vi "Puckbot Main.vi"() -> ()   [LabVIEW 2019]
uses:
  SubVIs/Voter Info.ctl
  Vote Handler/Vote Result.ctl
  Vote Handler/Vote Status Update.ctl
  SubVIs/References.ctl
  <vilib>/MediaMongrels Ltd/Message Queue Helper/ctl_QMH_Message_Typedef.ctl
  SubVIs/Move Type.ctl
  Vote Handler/VoteMessage.ctl
  LINX-PCA9865 PWM/LINX-PCA9865 PWM.lvclass
  LINX-PCA9865 PWM/LINX-PCA9865 PWM.lvclass/LINX-PCA9865 PWM.ctl
  LINX-PCA9865 PWM/Write LINX Resource.vi
  LINX-PCA9865 PWM/Write I2C Slave Address (0x40).vi
  LINX-PCA9865 PWM/Write LINX I2C Channel.vi
  LINX-PCA9865 PWM/Read LINX Resource.vi
  <vilib>/MakerHub/LINX/Public/Utilities/Open Local.vi
  <vilib>/MediaMongrels Ltd/WebSockets/Sockets/VISA TCP Listener/VISA TCP Listener.lvclass
  <vilib>/MediaMongrels Ltd/WebSockets/WebSockets/WebSocket Server/WebSocket Server.lvclass
  <vilib>/MediaMongrels Ltd/Message Queue Helper/MessageQueueHelper.lvlib
  <vilib>/MakerHub/LINX/LMH-LINX.lvlib
panel:
  out "Frequency (Hz)":dbl
  out "Error":errorcluster
  in  "stop":bool
  out "Drives Enabled?":bool
  out "Status":T1
  out "Time Remaining":dbl format="%<%H:%M:%S%2u>t"
  out "Vote Count":T2[](array[typedef])
  out "Voters":cluster{"VoterID":i32, "VoterInfo":T3}[](array[cluster])
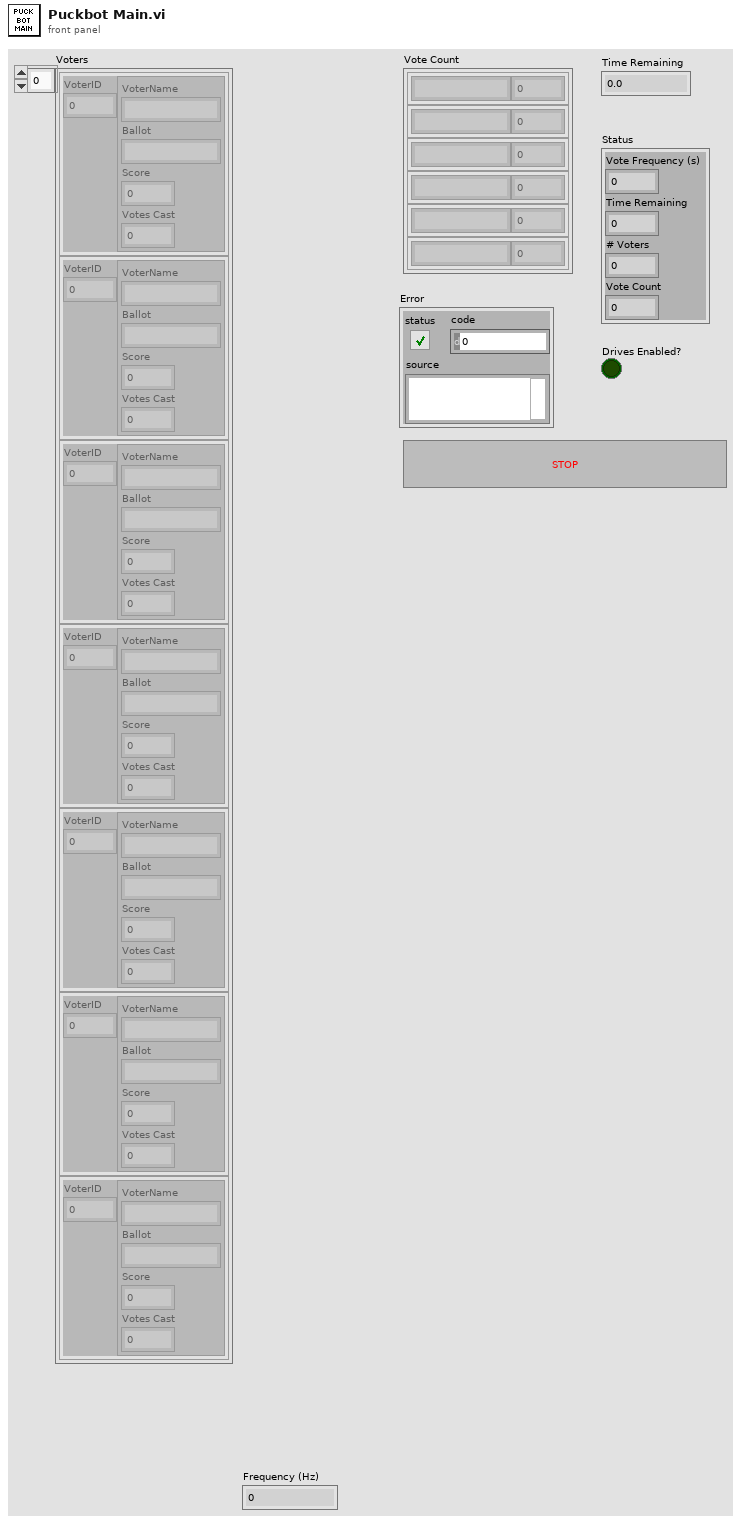
[diagram p1: front panel]
types:
  T1 = typedef "Vote Status Update.ctl" = cluster{"Vote Frequency (s)":dbl, "Time Remaining":dbl, "# Voters":i32, "Vote Count":i32}
  T2 = typedef "Vote Result.ctl" = cluster{"Vote":string, "Count":i32}
  T3 = typedef "Voter Info.ctl" = cluster{"VoterName":string, "Ballot":string, "Score":i32, "Votes Cast":i32}
  T4 = typedef "Move Type.ctl" = cluster{"Option":string, "Left":dbl, "Right":dbl, "Duration":dbl}
  T5 = typedef "References.ctl" = cluster{"Vote Queue":refnum<queue>, "Message Event":refnum<user-event>}
  T6 = typedef "LMH-LINX.lvlib/LINX Ref.ctl" = cluster{"IO":T7, "Interface":T8, "LINX Device Config":T9}
  T7 = typedef "LMH-LINX.lvlib/Platform.ctl" = enum16{"Remote", "Local"}
  T8 = typedef "LMH-LINX.lvlib/Interface.ctl" = enum16{"Serial", "TCP"}
  T9 = typedef "LMH-LINX.lvlib/Device.lvlib/LINX Device Config.ctl" = cluster{"Interface":T8, "COM Port":refnum<visa-resource-name>, "TCP Configuration":T10, "Device Family":u8, "Device ID":u8, "Device Name":string, "TCP Ref":refnum<k5>, "Channels":T11}
  T10 = typedef "LMH-LINX.lvlib/Device.lvlib/TCP Config.ctl" = cluster{"IP Address":string, "Port":u16}
  T11 = typedef "LMH-LINX.lvlib/Channels.ctl" = cluster{"DI":u8[], "DO":u8[], "AI":u8[], "AO":u8[], "PWM":u8[], "QE":u8[], "UART":u8[], "I2C 2":u8[], "SPI":u8[], "CAN":u8[], "Servo":u8[], "AI Ref (V)":dbl, "AI Resolution (Bits)":u8, "AO Ref (V)":dbl, "AO Resolution (Bits)":u8}
  T12 = enum16{"LED/PWM00", "LED/PWM01", "LED/PWM02", "LED/PWM03", "LED/PWM04", "LED/PWM05", "LED/PWM06", "LED/PWM07", "LED/PWM08", "LED/PWM09", "LED/PWM10", "LED/PWM11", "LED/PWM12", "LED/PWM13", "LED/PWM14", "LED/PWM15"}[]
  T13 = typedef "VoteMessage.ctl" = cluster{"VoterID":i32, "VoterInfo":T3}
  T14 = typedef "Scoreboard Entry.ctl" = cluster{"VoterName":string, "Score":i32}
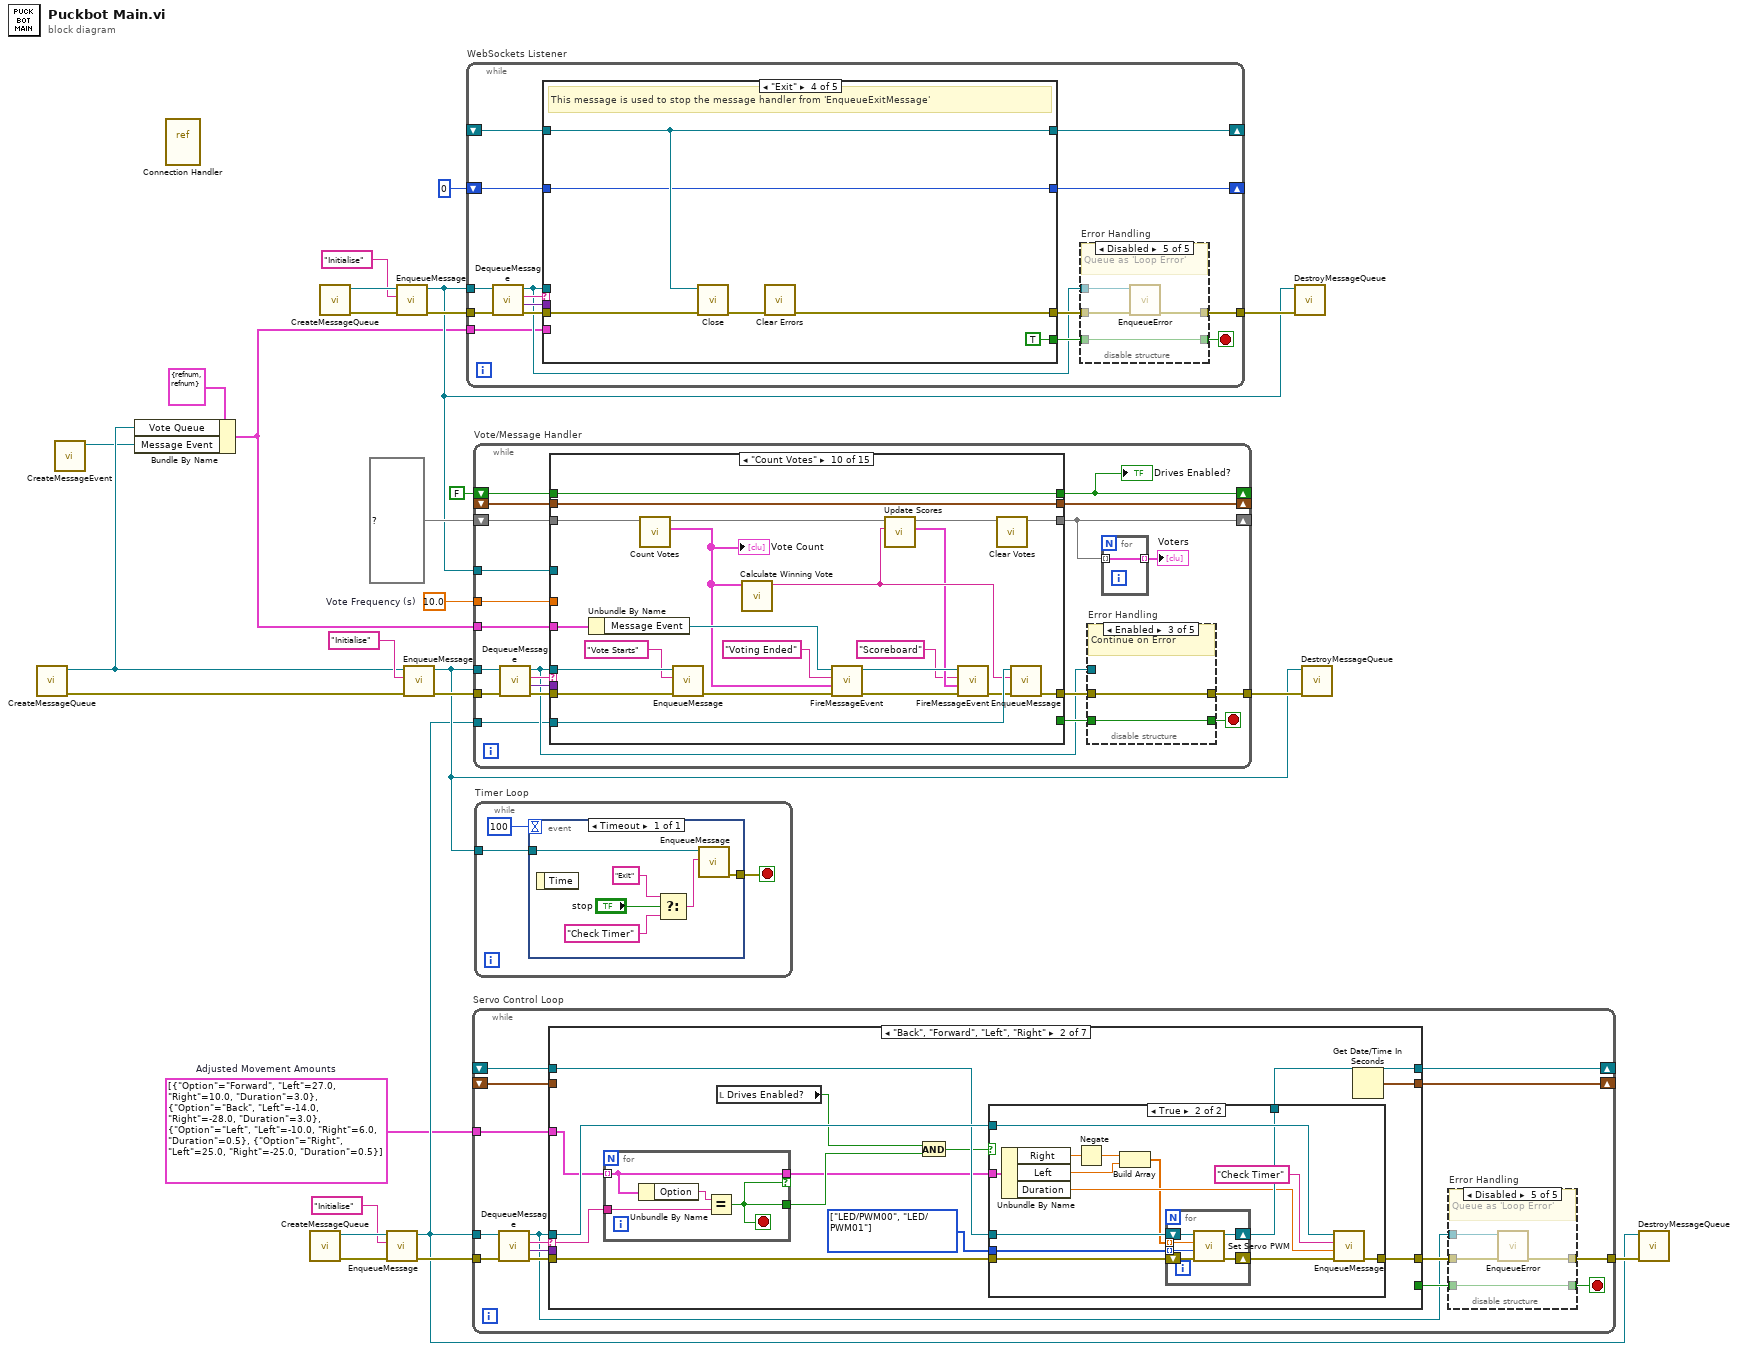
[diagram p0: block diagram]
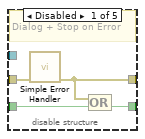
[diagram p2: hidden frame]
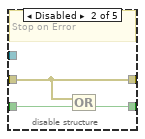
[diagram p3: hidden frame]
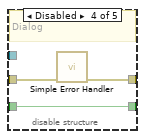
[diagram p5: hidden frame]
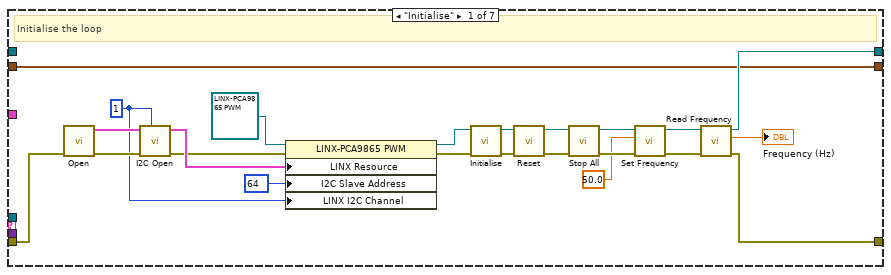
[diagram p6: hidden frame]
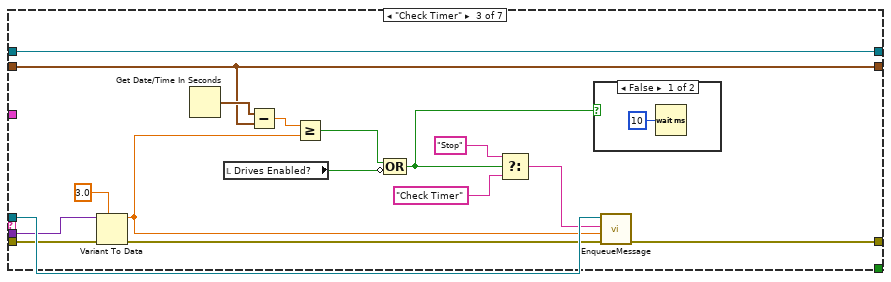
[diagram p8: hidden frame]
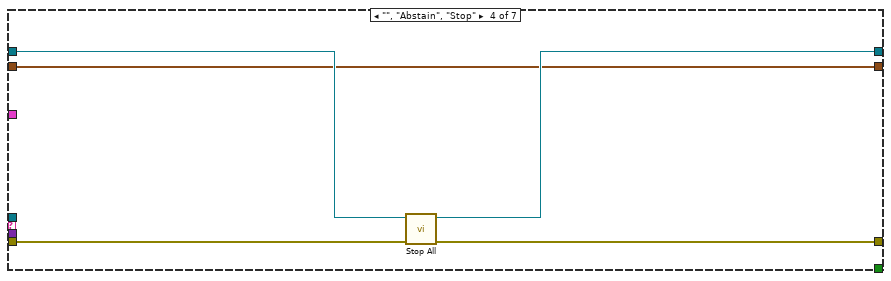
[diagram p10: hidden frame]
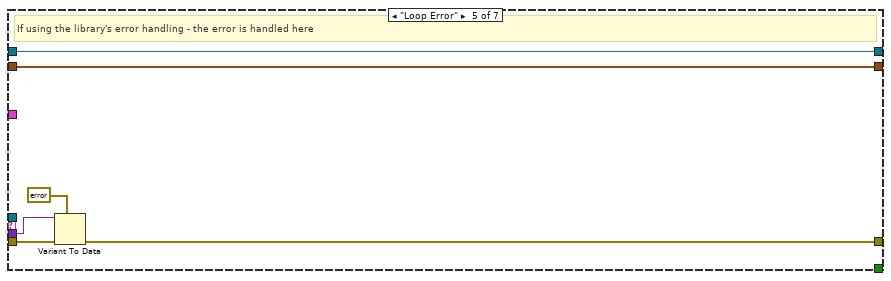
[diagram p11: hidden frame]
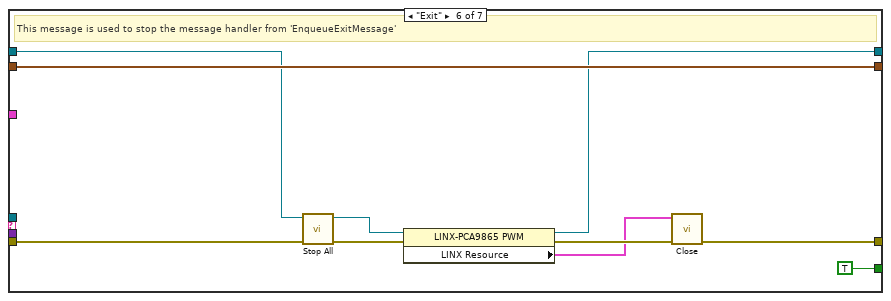
[diagram p12: hidden frame]
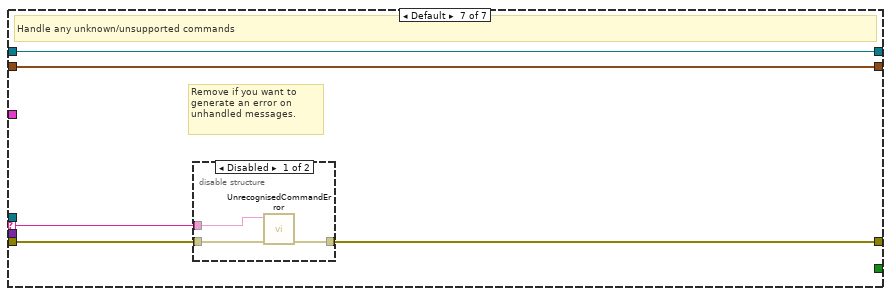
[diagram p13: hidden frame]
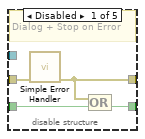
[diagram p15: hidden frame]
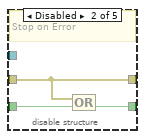
[diagram p16: hidden frame]
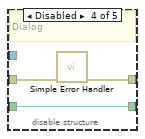
[diagram p17: hidden frame]
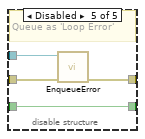
[diagram p18: hidden frame]
diagram:
  w1 = T4[] [{"Option"="Forward", "Left"=27.0, "Right"=10.0, "Duration"=3.0}, {"Option"="Back", "Left"=-14.0, "Right"=-28.0, "Duration"=3.0}, {"Option"="Left", "Left"=-10.0, "Right"=6.0, "Duration"=0.5}, {"Option"="Right", "Left"=25.0, "Right"=-25.0, "Duration"=0.5}]  # Adjusted Movement Amounts
  w14 = 10.0  # Vote Frequency (s)
  n1 = call <vilib>:"CreateMessageQueue.vi"() -> ("error out"=w17:errorcluster, "queue out"=w12:refnum<queue>)  [unwired: 9 in, 1 out]
  n2 = call <vilib>:"CreateMessageEvent.vi"() -> ("Message Event"=w11:refnum<user-event>)  [unwired: 10 in, 1 out]
  n3 = Bundle By Name(cluster=T5 {"Vote Queue"=refnum, "Message Event"=refnum} ("output cluster"), "Vote Queue"=w12, "Message Event"=w11) -> (w9:T5)
  n4 = vi-ref "Connection Handler.vi"() -> ()  [unwired: 1 out]
  n5 = call <vilib>:"CreateMessageQueue.vi"() -> ("error out"=w3:errorcluster, "queue out"=w5:refnum<queue>)  [unwired: 9 in, 1 out]
  n6 = call <vilib>:"CreateMessageQueue.vi"() -> ("error out"=w22:errorcluster, "queue out"=w24:refnum<queue>)  [unwired: 9 in, 1 out]
  n7 = call <vilib>:"EnqueueMessage.vi"("error in (no error)"=w3, "Command"="Initialise", "Message Queue in"=w5) -> ("error out"=w6:errorcluster, "Message Queue out"=w2:refnum<queue>)  [unwired: 6 in, 1 out]
  n8 = call <vilib>:"EnqueueMessage.vi"("error in (no error)"=w22, "Command"="Initialise", "Message Queue in"=w24) -> ("error out"=w25:errorcluster, "Message Queue out"=w10:refnum<queue>)  [unwired: 6 in, 1 out]
  n9 = call <vilib>:"EnqueueMessage.vi"("error in (no error)"=w17, "Command"="Initialise", "Message Queue in"=w12) -> ("error out"=w19:errorcluster, "Message Queue out"=w15:refnum<queue>)  [unwired: 6 in, 1 out]
  n10 = while "WebSockets Listener" {
    tunnel: w25 -> [w41]
    tunnel: w10 -> [w40]
    tunnel: [w33] -> w26
    shift-right: [w31] -> _
    shift-left: _ -> [w30]
    tunnel: w9 -> [w29]
    shift-right: [w27] -> _
    shift-left: 0 -> [w28]
    stop <- w35 stop-if-true
    n11 = call <vilib>:"DequeueMessage.vi"("error in (no error)"=w41, "Message Queue in"=w40) -> ("error out"=w37:errorcluster, "Data"=w38:variant, "Command"=w39:string, "Message Queue out"=w32:refnum<queue>)  [unwired: 5 in, 1 out]
    n12 = case shown="\"Exit\"" w39 {
      selector: w39 -> [_ _ _ _ w130]
      tunnel: w38 -> [_ _ w120 _ _]
      tunnel: w37 -> [w65 w84 w121 w126 w132]
      tunnel: w32 -> [w60 w78 _ _ _]
      tunnel: [w61 w79 w112 w125 w131] -> w36
      tunnel: [_ _ _ TRUE _] -> w34
      tunnel: [w66 w82 w118 w124 w129] -> w31
      tunnel: w30 -> [w64 w83 w118 w124 w129]
      tunnel: w29 -> [_ w77 w111 _ _]
      tunnel: w28 -> [w58 w76 w117 w123 w128]
      tunnel: [w58 w75 w117 w123 w128] -> w27
      frame "Initialise" {
        # "Initialise the loop"
        n13 = call-dynamic <vilib>:"Close.vi"("error in (no error)"=w65, "VISA TCP Listener in"=w64) -> ("error out"=w59:errorcluster)  [unwired: 9 in]
        n14 = call <vilib>:"Clear Errors.vi"("error in (no error)"=w59) -> ("error out"=w63:errorcluster)  [unwired: 5 in, 1 out]
        n15 = call <vilib>:"New VISA TCP Listener.vi"("error in (no error)"=w63) -> ("error out"=w68:errorcluster, "VISA TCP Listener out"=w67:refnum<class "VISA TCP Listener.lvclass">)  [unwired: 9 in]
        n16 = call-dynamic "Create Listener.vi"("error in (no error)"=w68, "Port"=u16 6123, "VISA TCP Listener in"=w67) -> ("error out"=w62:errorcluster, "VISA TCP Listener out"=w66:refnum<class "VISA TCP Listener.lvclass">)  [unwired: 7 in]
        n17 = case shown="No Error" w62 {
          selector: w62 -> [w73 w74]
          tunnel: [w72 w74] -> w61
          tunnel: w60 -> [w71 _]
          frame No Error {
            n18 = call <vilib>:"EnqueueMessage.vi"("error in (no error)"=w73, "Command"="Listen", "Message Queue in"=w71) -> ("error out"=w72:errorcluster)  [unwired: 6 in, 2 out]
          }
          frame Error {
          }
        }
      }
      frame "Listen" {
        n19 = call-dynamic "Wait on Listener.vi"("error in (no error)"=w84, "timeout ms (5000)"=200, "VISA TCP Listener in"=w83) -> ("error out"=w81:errorcluster, "Socket out"=w80:refnum<class "Socket.lvclass">, "VISA TCP Listener out"=w82:refnum<class "VISA TCP Listener.lvclass">)  [unwired: 6 in]
        n20 = case shown="No Error" w81 {
          selector: w81 -> [w96 w102 w108]
          tunnel: w80 -> [w97 _ _]
          tunnel: [w90 w102 w106] -> w79
          tunnel: w78 -> [w92 _ w105]
          tunnel: w77 -> [w88 _ _]
          tunnel: w76 -> [w87 w100 w103]
          tunnel: [w86 w100 w103] -> w75
          frame No Error {
            n21 = call <vilib>:"New Server from Socket.vi"("error in (no error)"=w96, "Socket"=w97) -> ("error out"=w98:errorcluster, "WebSocket Server out"=w99:refnum<class "WebSocket Server.lvclass">)  [unwired: 8 in]
            n22 = call-dynamic "Handshake.vi"("error in (no error)"=w98, "WebSocket Connection in"=w99) -> ("error out"=w95:errorcluster, "WebSocket Connection out"=w94:refnum<class "WebSocket Server.lvclass">)  [unwired: 8 in]
            n23 = call "Launch Connection Handler.vi"("error in (no error)"=w95, "ConnectionID"=w87, "References in"=w88, "WebSocket Connection in"=w94) -> ("error out"=w93:errorcluster)  [unwired: 7 in]
            n24 = call <vilib>:"EnqueueMessage.vi"("Command"="Listen", "Message Queue in"=w92) -> ("error out"=w89:errorcluster)  [unwired: 7 in, 2 out]
            n25 = Increment(x=w87) -> (x+1=w86:i32)
            n26 = Merge Errors(w93, w89) -> (w90:errorcluster)
          }
          frame Default {
            n27 = Wait (ms)(milliseconds to wait=u32 10) -> ()  [unwired: 1 out]
          }
          frame Error {
            n28 = call <vilib>:"Clear Errors.vi"("error in (no error)"=w108) -> ("error out"=w107:errorcluster)  [unwired: 5 in, 1 out]
            n29 = call <vilib>:"EnqueueMessage.vi"("error in (no error)"=w107, "Command"="Listen", "Message Queue in"=w105) -> ("error out"=w106:errorcluster)  [unwired: 6 in, 2 out]
          }
        }
      }
      frame "Loop Error" {
        # "If using the library's error handling - the error is handled here"
        n30 = Variant To Data(error in=w121, type=errorcluster {"status"=FALSE, "code"=0, "source"=""} ("error constant"), Variant=w120) -> (data=w114:errorcluster, error out=w116:errorcluster)
        n31 = Unbundle By Name(w111) -> ("Vote Queue"=w110:refnum<queue>)
        n32 = Merge Errors(w114, w116) -> (w115:errorcluster)
        n33 = call <vilib>:"EnqueueError.vi"("Source"="Listener", "error in (no error)"=w115, "Message Queue in"=w110) -> ("error out"=w113:errorcluster)  [unwired: 8 in]
        n34 = call <vilib>:"Clear Errors.vi"("error in (no error)"=w113) -> ("error out"=w112:errorcluster)  [unwired: 5 in, 1 out]
      }
      frame "Exit" {
        # "This message is used to stop the message handler from 'EnqueueExitMessage'"
        n35 = call-dynamic <vilib>:"Close.vi"("error in (no error)"=w126, "VISA TCP Listener in"=w124) -> ("error out"=w122:errorcluster)  [unwired: 9 in]
        n36 = call <vilib>:"Clear Errors.vi"("error in (no error)"=w122) -> ("error out"=w125:errorcluster)  [unwired: 5 in, 1 out]
      }
      frame Default {
        # "Remove if you want to generate an error on unhandled messages."
        # "Handle any unknown/unsupported commands"
        n37 = disable-structure shown="Disabled" {
          disable-tunnel: w132 -> [w134 w136]
          disable-tunnel: [w135 w136] -> w131
          disable-tunnel: w130 -> [w133 _]
          frame Disabled {
            n38 = call <vilib>:"UnrecognisedCommandError.vi"("error in (no error)"=w134, "Command"=w133) -> ("error out"=w135:errorcluster)  [unwired: 9 in]
          }
          frame Enabled {
          }
        }
      }
    }
    n39 = disable-structure "Error Handling" shown="Disabled" {
      disable-tunnel: w34 -> [w45 w48 w49 w52 w55]
      disable-tunnel: w36 -> [w44 w46 w50 w53 w57]
      disable-tunnel: [w43 w47 w49 w52 w55] -> w35
      disable-tunnel: [w42 w46 w50 w51 w56] -> w33
      disable-tunnel: w32 -> [_ _ _ _ w54]
      frame Disabled {
        # "Dialog + Stop on Error"
        n40 = call <vilib>:"Simple Error Handler.vi"("error in (no error)"=w44) -> ("error out"=w42:errorcluster)  [unwired: 4 in, 4 out]
        n41 = Compound Arithmetic op=OR(w42, w45) -> (w43:bool)
      }
      frame Disabled {
        # "Stop on Error"
        n42 = Compound Arithmetic op=OR(w46, w48) -> (w47:bool)
      }
      frame Enabled {
        # "Continue on Error"
      }
      frame Disabled {
        # "Dialog"
        n43 = call <vilib>:"Simple Error Handler.vi"("error in (no error)"=w53) -> ("error out"=w51:errorcluster)  [unwired: 4 in, 4 out]
      }
      frame Disabled {
        # "Queue as 'Loop Error'"
        n44 = call <vilib>:"EnqueueError.vi"("error in (no error)"=w57, "Message Queue in"=w54) -> ("error out"=w56:errorcluster)  [unwired: 9 in]
      }
    }
  }
  n45 = while "Servo Control Loop" {
    tunnel: w6 -> [w151]
    tunnel: w2 -> [w150]
    tunnel: [w143] -> w7
    shift-right: [w141] -> _
    shift-left: _ -> [w140]
    shift-right: [w139] -> _
    shift-left: _ -> [w138]
    tunnel: w1 -> [w137]
    stop <- w145 stop-if-true
    n46 = call <vilib>:"DequeueMessage.vi"("error in (no error)"=w151, "Message Queue in"=w150) -> ("error out"=w147:errorcluster, "Data"=w148:variant, "Command"=w149:string, "Message Queue out"=w142:refnum<queue>)  [unwired: 5 in, 1 out]
    n47 = case shown="\"Back\", \"Forward\", \"Left\", \"Right\"" w149 {
      selector: w149 -> [_ w193 _ _ _ _ w271]
      tunnel: w148 -> [_ _ w232 _ w256 _ _]
      tunnel: w147 -> [w170 w199 w239 w252 w258 w266 w273]
      tunnel: w142 -> [_ w201 w240 _ _ _ _]
      tunnel: [w169 w202 w238 w251 w257 w260 w272] -> w146
      tunnel: [_ _ _ _ _ TRUE _] -> w144
      tunnel: [w171 w197 w246 w249 w254 w263 w270] -> w141
      tunnel: w140 -> [_ w198 w246 w250 w254 w265 w270]
      tunnel: [w168 w203 w244 w248 w253 w267 w269] -> w139
      tunnel: w138 -> [w168 _ w244 w248 w253 w267 w269]
      tunnel: w137 -> [_ w192 _ _ _ _ _]
      frame "Initialise" {
        w174 = u8 1 ("I2C Channel")
        # "Initialise the loop"
        n48 = call-poly <vilib>:"Open.vi"("Error In"=w170) -> ("Error Out"=w177:errorcluster, "LINX Resource"=w176:T6)  [unwired: 8 in, 1 out]
        n49 = call <vilib>:"I2C Open.vi"("I2C Channel (0)"=w174, "Error In"=w177, "LINX Resource"=w176) -> ("Error Out"=w178:errorcluster, "LINX Resource"=w179:T6)  [unwired: 7 in]
        n50 = property class="LINX-PCA9865 PWM"(reference=refnum<class "LINX-PCA9865 PWM.lvclass"> refnum ("LINX-PCA9865 PWM.lvclass"), error in=w178, "LINX Resource"=w179, "I2C Slave Address"=u8 64 ("I2C Slave Address (0)"), "LINX I2C Channel"=w174) -> (reference out=w181:refnum<class "LINX-PCA9865 PWM.lvclass">, error out=w180:errorcluster)
        n51 = call-dynamic "Initialise.vi"("error in (no error)"=w180, "PWM in"=w181) -> ("error out"=w184:errorcluster, "PWM out"=w183:refnum<class "LINX-PCA9865 PWM.lvclass">)  [unwired: 8 in]
        n52 = call-dynamic "Reset.vi"("error in (no error)"=w184, "PWM in"=w183) -> ("error out"=w185:errorcluster, "PWM out"=w186:refnum<class "LINX-PCA9865 PWM.lvclass">)  [unwired: 8 in]
        n53 = call-dynamic "Stop All.vi"("error in (no error)"=w185, "LINX-PCA9865 PWM in"=w186) -> ("error out"=w189:errorcluster, "LINX-PCA9865 PWM out"=w190:refnum<class "LINX-PCA9865 PWM.lvclass">)  [unwired: 8 in]
        n54 = call-dynamic "Set Frequency.vi"("error in (no error)"=w189, "Frequency (1000Hz)"=50.0, "PWM in"=w190) -> ("error out"=w187:errorcluster, "PWM out"=w188:refnum<class "LINX-PCA9865 PWM.lvclass">)  [unwired: 7 in]
        n55 = call-dynamic "Read Frequency.vi"("error in (no error)"=w187, "PWM in"=w188) -> ("error out"=w169:errorcluster, "Frequency (Hz)"=→"Frequency (Hz)":dbl, "PWM out"=w171:refnum<class "LINX-PCA9865 PWM.lvclass">)  [unwired: 7 in]
      }
      frame "Back", "Forward", "Left", "Right" {
        w200 = T12 [enum."LED/PWM00", enum."LED/PWM01"] items=["LED/PWM00", "LED/PWM01", "LED/PWM02", "LED/PWM03", "LED/PWM04", "LED/PWM05", "LED/PWM06", "LED/PWM07", "LED/PWM08", "LED/PWM09", "LED/PWM10", "LED/PWM11", "LED/PWM12", "LED/PWM13", "LED/PWM14", "LED/PWM15"] ("LEDn (PWM channel)")
        n56 = for {
          tunnel: w192 -> [w206] mode=indexing
          tunnel: [w206] -> w191 if=w204
          tunnel: w193 -> [w205]
          tunnel: [w204] -> w195
          stop <- w204 stop-if-true
          n57 = Unbundle By Name(w206) -> ("Option"=w207:string)
          n58 = Equal?(x=w207, y=w205) -> (x = y?=w204:bool)
        }
        n59 = local read "Drives Enabled?"() -> (w196:bool)
        n60 = And(x=w196, y=w195) -> (x .and. y?=w194:bool)
        n61 = case shown="True" w194 {
          tunnel: [w208 w223] -> w202
          tunnel: w201 -> [_ w222]
          tunnel: w200 -> [_ w220]
          tunnel: w199 -> [w208 w219]
          tunnel: w198 -> [w209 w217]
          tunnel: [w209 w216] -> w197
          tunnel: w191 -> [_ w211]
          frame False {
          }
          frame True {
            n62 = Unbundle By Name(w211) -> ("Right"=w213:dbl, "Left"=w214:dbl, "Duration"=w212:dbl)
            n63 = Negate(x=w213) -> (-x=w215:dbl)
            n64 = Build Array(w215, w214) -> (w210:dbl[])
            n65 = for {
              tunnel: w210 -> [w226] mode=indexing
              tunnel: w220 -> [w225] mode=indexing
              shift-right: [w227] -> w216
              shift-left: w217 -> [w229]
              shift-right: [w228] -> w218
              shift-left: w219 -> [w224]
              n66 = call "Set Servo PWM.vi"("error in (no error)"=w224, "LEDn (PWM channel)"=w225, "Servo Speed (-100 to 100%)"=w226, "LINX-PCA9865 PWM in"=w229) -> ("error out"=w228:errorcluster, "LINX-PCA9865 PWM out"=w227:refnum<class "LINX-PCA9865 PWM.lvclass">)  [unwired: 6 in]
            }
            n67 = call <vilib>:"EnqueueMessage.vi"("error in (no error)"=w218, "Data"=w212, "Command"="Check Timer", "Message Queue in"=w222) -> ("error out"=w223:errorcluster)  [unwired: 5 in, 2 out]
          }
        }
        n68 = Get Date/Time In Seconds() -> (seconds since 1Jan1904=w203:timestamp)
      }
      frame "Check Timer" {
        n69 = Variant To Data(error in=w239, type=3.0 ("y"), Variant=w232) -> (data=w230:dbl, error out=w233:errorcluster)
        n70 = Get Date/Time In Seconds() -> (seconds since 1Jan1904=w245:timestamp)
        n71 = local read "Drives Enabled?"() -> (w241:bool)
        n72 = Subtract(x=w245, y=w244) -> (x-y=w243:dbl)
        n73 = Greater Or Equal?(x=w243, y=w230) -> (x >= y?=w242:bool)
        n74 = Compound Arithmetic op=OR(w242, invert w241) -> (w234:bool)
        n75 = Select(t="Stop", s=w234, f="Check Timer") -> (s? t:f=w235:string)
        n76 = case shown="False" w234 {
          frame False {
            n77 = Wait (ms)(milliseconds to wait=u32 10) -> ()  [unwired: 1 out]
          }
          frame True {
          }
        }
        n78 = call <vilib>:"EnqueueMessage.vi"("error in (no error)"=w233, "Data"=w230, "Command"=w235, "Message Queue in"=w240) -> ("error out"=w238:errorcluster)  [unwired: 5 in, 2 out]
      }
      frame "", "Abstain", "Stop" {
        n79 = call-dynamic "Stop All.vi"("error in (no error)"=w252, "LINX-PCA9865 PWM in"=w250) -> ("error out"=w251:errorcluster, "LINX-PCA9865 PWM out"=w249:refnum<class "LINX-PCA9865 PWM.lvclass">)  [unwired: 8 in]
      }
      frame "Loop Error" {
        # "If using the library's error handling - the error is handled here"
        n80 = Variant To Data(error in=w258, type=errorcluster {"status"=FALSE, "code"=0, "source"=""} ("error constant"), Variant=w256) -> (error out=w257:errorcluster)  [unwired: 1 out]
      }
      frame "Exit" {
        # "This message is used to stop the message handler from 'EnqueueExitMessage'"
        n81 = call-dynamic "Stop All.vi"("error in (no error)"=w266, "LINX-PCA9865 PWM in"=w265) -> ("error out"=w262:errorcluster, "LINX-PCA9865 PWM out"=w264:refnum<class "LINX-PCA9865 PWM.lvclass">)  [unwired: 8 in]
        n82 = property class="LINX-PCA9865 PWM"(reference=w264, error in=w262) -> (reference out=w263:refnum<class "LINX-PCA9865 PWM.lvclass">, error out=w261:errorcluster, "LINX Resource"=w259:T6)
        n83 = call <vilib>:"Close.vi"("Error In"=w261, "LINX Resource"=w259) -> ("Error Out"=w260:errorcluster)  [unwired: 9 in]
      }
      frame Default {
        # "Remove if you want to generate an error on unhandled messages."
        # "Handle any unknown/unsupported commands"
        n84 = disable-structure shown="Disabled" {
          disable-tunnel: w273 -> [w275 w277]
          disable-tunnel: [w276 w277] -> w272
          disable-tunnel: w271 -> [w274 _]
          frame Disabled {
            n85 = call <vilib>:"UnrecognisedCommandError.vi"("error in (no error)"=w275, "Command"=w274) -> ("error out"=w276:errorcluster)  [unwired: 9 in]
          }
          frame Enabled {
          }
        }
      }
    }
    n86 = disable-structure "Error Handling" shown="Disabled" {
      disable-tunnel: w144 -> [w155 w158 w159 w162 w165]
      disable-tunnel: w146 -> [w154 w156 w160 w163 w167]
      disable-tunnel: [w153 w157 w159 w162 w165] -> w145
      disable-tunnel: [w152 w156 w160 w161 w166] -> w143
      disable-tunnel: w142 -> [_ _ _ _ w164]
      frame Disabled {
        # "Dialog + Stop on Error"
        n87 = call <vilib>:"Simple Error Handler.vi"("error in (no error)"=w154) -> ("error out"=w152:errorcluster)  [unwired: 4 in, 4 out]
        n88 = Compound Arithmetic op=OR(w152, w155) -> (w153:bool)
      }
      frame Disabled {
        # "Stop on Error"
        n89 = Compound Arithmetic op=OR(w156, w158) -> (w157:bool)
      }
      frame Enabled {
        # "Continue on Error"
      }
      frame Disabled {
        # "Dialog"
        n90 = call <vilib>:"Simple Error Handler.vi"("error in (no error)"=w163) -> ("error out"=w161:errorcluster)  [unwired: 4 in, 4 out]
      }
      frame Disabled {
        # "Queue as 'Loop Error'"
        n91 = call <vilib>:"EnqueueError.vi"("error in (no error)"=w167, "Message Queue in"=w164) -> ("error out"=w166:errorcluster)  [unwired: 9 in]
      }
    }
  }
  n92 = while "Vote/Message Handler" {
    tunnel: w19 -> [w298]
    tunnel: w15 -> [w297]
    tunnel: [w290] -> w20
    shift-right: [w287] -> _
    shift-left: map{i32, T3} {} ("map") -> [w288]
    tunnel: w14 -> [w285]
    shift-right: [w284] -> _
    shift-left: _ -> [w283]
    tunnel: w9 -> [w282]
    tunnel: w10 -> [w281]
    shift-right: [w280] -> _
    shift-left: FALSE -> [w279]
    tunnel: w2 -> [w278]
    stop <- w292 stop-if-true
    n93 = call <vilib>:"DequeueMessage.vi"("error in (no error)"=w298, "Message Queue in"=w297) -> ("error out"=w294:errorcluster, "Data"=w295:variant, "Command"=w296:string, "Message Queue out"=w289:refnum<queue>)  [unwired: 5 in, 1 out]
    n94 = case shown="\"Count Votes\"" w296 {
      selector: w296 -> [_ _ _ _ _ _ _ _ _ _ _ _ _ _ w476]
      tunnel: w295 -> [_ _ w335 w351 w360 _ _ _ _ _ _ w451 w458 _ _]
      tunnel: w294 -> [w319 w323 w337 w353 w362 w366 w374 w389 w404 w437 w441 w452 w460 w466 w478]
      tunnel: w289 -> [_ _ w327 _ _ _ _ w387 _ w429 _ _ _ _ _]
      tunnel: [w319 w323 w328 w352 w361 w366 w372 w388 w403 w426 w441 w445 w459 w468 w477] -> w293
      tunnel: [_ _ _ _ _ _ _ _ _ _ _ _ _ TRUE _] -> w291
      tunnel: w288 -> [w318 w322 w326 w349 w359 w365 w373 w380 w407 w435 w440 w448 w456 w471 w475]
      tunnel: [w318 w322 w332 w348 w358 w365 w373 w380 w407 w423 w440 w448 w456 w471 w475] -> w287
      tunnel: w285 -> [_ _ _ _ _ _ _ w382 w410 _ _ _ _ _ _]
      tunnel: [w317 w321 w329 w344 w357 w364 w368 w391 w413 w436 w439 w450 w455 w470 w474] -> w284
      tunnel: w283 -> [w317 w321 w329 w344 w357 w364 _ w390 w413 w436 w439 w450 w455 w470 w474]
      tunnel: w282 -> [_ _ _ _ _ _ w371 _ w402 w433 _ w446 _ w465 _]
      tunnel: w281 -> [_ _ _ _ _ _ _ _ _ _ _ _ _ w469 _]
      tunnel: [w316 w320 w324 w343 w354 w363 w367 w375 w398 w427 w438 w442 w454 w467 w473] -> w280
      tunnel: w279 -> [w316 w320 w324 w343 w354 w363 w367 w375 w398 w427 w438 _ w454 w467 w473]
      tunnel: w278 -> [_ _ _ _ _ _ _ _ _ w425 _ _ _ w461 _]
      frame "Initialise" {
        # "Initialise the loop"
      }
      frame "-- Voter Registration --" {
      }
      frame "Register Voter" {
        # "New voter has connected - add to the map"
        n95 = Variant To Data(error in=w337, type=T13 {"VoterID"=0, "VoterInfo"={"VoterName"="", "Ballot"="", "Score"=0, "Votes Cast"=0}}, Variant=w335) -> (data=w333:T13, error out=w336:errorcluster)
        n96 = Unbundle By Name(w333) -> ("VoterID"=w331:i32, "VoterInfo"=w330:T3)
        n97 = call "Register Voter.vi"("VoterInfo"=w330, "VoterID"=w331, "map in"=w326) -> ("map out"=w332:map{i32, T3})  [unwired: 8 in]
        n98 = Empty Collection?(1:w326) -> (0:w325:bool)
        n99 = case shown="True" w325 {
          tunnel: w336 -> [w338 w342]
          tunnel: [w338 w341] -> w328
          tunnel: w327 -> [_ w340]
          frame False {
          }
          frame True {
            n100 = call <vilib>:"EnqueueMessage.vi"("error in (no error)"=w342, "Command"="Vote Starts", "Message Queue in"=w340) -> ("error out"=w341:errorcluster)  [unwired: 6 in, 2 out]
          }
        }
      }
      frame "Vote" {
        # "Voter has cast their vote- update the map"
        n101 = Variant To Data(error in=w353, type=T13 {"VoterID"=0, "VoterInfo"={"VoterName"="", "Ballot"="", "Score"=0, "Votes Cast"=0}}, Variant=w351) -> (data=w347:T13, error out=w352:errorcluster)
        n102 = Unbundle By Name(w347) -> ("VoterID"=w346:i32, "VoterInfo"=w345:T3)
        n103 = call "Vote.vi"("VoterInfo"=w345, "VoterID"=w346, "map in"=w349) -> ("map out"=w348:map{i32, T3})  [unwired: 8 in]
      }
      frame "Deregister Voter" {
        # "Voter disconnected - remove from map"
        n104 = Variant To Data(error in=w362, type=0 ("VoterID"), Variant=w360) -> (data=w355:i32, error out=w361:errorcluster)
        n105 = Remove From Map(10:w355, 11:w359) -> (3:w358:map{i32, T3})  [unwired: 2 out]
      }
      frame "-- Vote Handling --" {
      }
      frame "Vote Starts" {
        n106 = Unbundle By Name(w371) -> ("Message Event"=w370:refnum<user-event>)
        n107 = call <vilib>:"FireMessageEvent.vi"("error in (no error)"=w374, "Command"="Vote Starts", "Message Event in"=w370) -> ("error out"=w372:errorcluster)  [unwired: 7 in, 1 out]
        n108 = Get Date/Time In Seconds() -> (seconds since 1Jan1904=w368:timestamp)
      }
      frame "Check Timer" {
        # "Check the time left to vote"
        n109 = Get Date/Time In Seconds() -> (seconds since 1Jan1904=w392:timestamp)
        n110 = Subtract(x=w392, y=w390) -> (x-y=w381:dbl)
        n111 = Subtract(x=w382, y=w381) -> (x-y=w378:dbl)
        n112 = Greater Or Equal?(x=w381, y=w382) -> (x >= y?=w384:bool)
        n113 = Max & Min(x=w378, y=0.0) -> (max(x,y)=→"Time Remaining":dbl)  [unwired: 1 out]
        n114 = Select(t=w392, s=w384, f=w390) -> (s? t:f=w391:timestamp)
        n115 = Empty Collection?(1:w380) -> (0:w379:bool)
        n116 = Select(t="Count Votes", s=w384, f="Send Update") -> (s? t:f=w385:string)
        n117 = case shown="False" w379 {
          tunnel: w389 -> [w396 w397]
          tunnel: [w395 w397] -> w388
          tunnel: w387 -> [w394 _]
          tunnel: w385 -> [w393 _]
          frame False {
            n118 = call <vilib>:"EnqueueMessage.vi"("error in (no error)"=w396, "Command"=w393, "Message Queue in"=w394) -> ("error out"=w395:errorcluster)  [unwired: 6 in, 2 out]
          }
          frame True {
          }
        }
      }
      frame "Send Update" {
        # "Sends an update to the electorate"
        n119 = Get Date/Time In Seconds() -> (seconds since 1Jan1904=w415:timestamp)
        n120 = Unbundle By Name(w402) -> ("Message Event"=w401:refnum<user-event>)
        n121 = Subtract(x=w415, y=w413) -> (x-y=w414:dbl)
        n122 = Subtract(x=w410, y=w414) -> (x-y=w411:dbl)
        n123 = Max & Min(x=w411, y=0.0) -> (max(x,y)=w409:dbl)  [unwired: 1 out]
        n124 = Collection Size(1:w407) -> (0:w408:i32)
        n125 = call "Votes Cast Count.vi"("map"=w407) -> ("Vote Count"=w406:i32)  [unwired: 10 in]
        n126 = Bundle(cluster=T1 {"Vote Frequency (s)"=0.0, "Time Remaining"=0.0, "# Voters"=0, "Vote Count"=0}, "Vote Frequency (s)"=w410, "Time Remaining"=w409, "# Voters"=w408, "Vote Count"=w406) -> (w400:T1)
        "Status" <- w400
        n127 = call <vilib>:"FireMessageEvent.vi"("error in (no error)"=w404, "Data"=w400, "Command"="Vote Status", "Message Event in"=w401) -> ("error out"=w403:errorcluster)  [unwired: 6 in, 1 out]
      }
      frame "Count Votes" {
        n128 = Unbundle By Name(w433) -> ("Message Event"=w431:refnum<user-event>)
        n129 = call "Count Votes.vi"("map in"=w435) -> ("Vote Count"=w424:T2[], "map out"=w434:map{i32, T3})  [unwired: 9 in]
        "Vote Count" <- w424
        n130 = call <vilib>:"EnqueueMessage.vi"("error in (no error)"=w437, "Command"="Vote Starts", "Message Queue in"=w429) -> ("error out"=w430:errorcluster)  [unwired: 6 in, 2 out]
        n131 = call "Calculate Winning Vote.vi"("Vote Count"=w424) -> ("Vote"=w421:string)  [unwired: 10 in]
        n132 = call <vilib>:"FireMessageEvent.vi"("error in (no error)"=w430, "Data"=w424, "Command"="Voting Ended", "Message Event in"=w431) -> ("error out"=w417:errorcluster, "Message Event out"=w420:refnum<user-event>)  [unwired: 6 in]
        n133 = call "Update Scores.vi"("Winning Vote"=w421, "map in"=w434) -> ("Score Table"=w419:T14[], "map out"=w422:map{i32, T3})  [unwired: 8 in]
        n134 = call <vilib>:"FireMessageEvent.vi"("error in (no error)"=w417, "Data"=w419, "Command"="Scoreboard", "Message Event in"=w420) -> ("error out"=w416:errorcluster)  [unwired: 6 in, 1 out]
        n135 = call "Clear Votes.vi"("map in"=w422) -> ("map out"=w423:map{i32, T3})  [unwired: 10 in]
        n136 = call <vilib>:"EnqueueMessage.vi"("error in (no error)"=w416, "Command"=w421, "Message Queue in"=w425) -> ("error out"=w426:errorcluster)  [unwired: 6 in, 2 out]
      }
      frame "-- Framework Messages --" {
      }
      frame "Enable Drives" {
        # "New voter has connected - add to the map"
        n137 = Variant To Data(error in=w452, type=FALSE, Variant=w451) -> (data=w442:bool, error out=w449:errorcluster)
        n138 = Unbundle By Name(w446) -> ("Message Event"=w444:refnum<user-event>)
        n139 = call <vilib>:"FireMessageEvent.vi"("error in (no error)"=w449, "Data"=w442, "Command"="Drive Status", "Message Event in"=w444) -> ("error out"=w445:errorcluster)  [unwired: 6 in, 1 out]
      }
      frame "Loop Error" {
        # "If using the library's error handling - the error is handled here"
        n140 = Variant To Data(error in=w460, type=errorcluster {"status"=FALSE, "code"=0, "source"=""} ("error constant"), Variant=w458) -> (data=→"Error":errorcluster, error out=w459:errorcluster)
      }
      frame "Exit" {
        # "This message is used to stop the message handler from 'EnqueueExitMessage'"
        n141 = Unbundle By Name(w465) -> ("Message Event"=w464:refnum<user-event>)
        n142 = call <vilib>:"FireExitEvent.vi"("error in (no error)"=w466, "Message Event in"=w464) -> ("error out"=w463:errorcluster)  [unwired: 8 in, 1 out]
        n143 = call <vilib>:"EnqueueExitMessage.vi"("error in (no error)"=w463, "Message Queue in"=w461) -> ("error out"=w462:errorcluster)  [unwired: 7 in, 2 out]
        n144 = call <vilib>:"EnqueueExitMessage.vi"("error in (no error)"=w462, "Message Queue in"=w469) -> ("error out"=w468:errorcluster)  [unwired: 7 in, 2 out]
      }
      frame Default {
        # "Remove if you want to generate an error on unhandled messages."
        # "Handle any unknown/unsupported commands"
        n145 = disable-structure shown="Disabled" {
          disable-tunnel: w478 -> [w480 w482]
          disable-tunnel: [w481 w482] -> w477
          disable-tunnel: w476 -> [w479 _]
          frame Disabled {
            n146 = call <vilib>:"UnrecognisedCommandError.vi"("error in (no error)"=w480, "Command"=w479) -> ("error out"=w481:errorcluster)  [unwired: 9 in]
          }
          frame Enabled {
          }
        }
      }
    }
    "Drives Enabled?" <- w280
    n147 = disable-structure "Error Handling" shown="Enabled" {
      disable-tunnel: w291 -> [w303 w306 w307 w310 w313]
      disable-tunnel: w293 -> [w302 w304 w308 w311 w315]
      disable-tunnel: [w301 w305 w307 w310 w313] -> w292
      disable-tunnel: [w300 w304 w308 w309 w314] -> w290
      disable-tunnel: w289 -> [_ _ _ _ w312]
      frame Disabled {
        # "Dialog + Stop on Error"
        n148 = call <vilib>:"Simple Error Handler.vi"("error in (no error)"=w302) -> ("error out"=w300:errorcluster)  [unwired: 4 in, 4 out]
        n149 = Compound Arithmetic op=OR(w300, w303) -> (w301:bool)
      }
      frame Disabled {
        # "Stop on Error"
        n150 = Compound Arithmetic op=OR(w304, w306) -> (w305:bool)
      }
      frame Enabled {
        # "Continue on Error"
      }
      frame Disabled {
        # "Dialog"
        n151 = call <vilib>:"Simple Error Handler.vi"("error in (no error)"=w311) -> ("error out"=w309:errorcluster)  [unwired: 4 in, 4 out]
      }
      frame Disabled {
        # "Queue as 'Loop Error'"
        n152 = call <vilib>:"EnqueueError.vi"("error in (no error)"=w315, "Message Queue in"=w312) -> ("error out"=w314:errorcluster)  [unwired: 9 in]
      }
    }
    n153 = for {
      tunnel: w287 -> [w299] mode=indexing
      tunnel: [w299] -> w286 mode=indexing
    }
    "Voters" <- w286
  }
  n154 = while "Timer Loop" {
    tunnel: w15 -> [w484]
    stop <- w483 stop-if-true
    n155 = event shown="[0] Timeout" {
      selector: _ -> [_]
      dyn-events: _ -> [_]
      timeout: 100 -> [_]
      tunnel: w484 -> [w491]
      tunnel: [w490] -> w483
      event Timeout {
        n156 = event-data() -> ()  [unwired: 1 in, 1 out]
        n157 = Select(t="Exit" ("Command"), s="stop", f="Check Timer" ("Command")) -> (s? t:f=w486:string)
        n158 = call <vilib>:"EnqueueMessage.vi"("Command"=w486, "Message Queue in"=w491) -> ("error out"=w490:errorcluster)  [unwired: 7 in, 2 out]
      }
    }
  }
  n159 = call <vilib>:"DestroyMessageQueue.vi"("error in (no error)"=w26, "Message Queue in"=w10) -> ()  [unwired: 9 in, 1 out]
  n160 = call <vilib>:"DestroyMessageQueue.vi"("error in (no error)"=w20, "Message Queue in"=w15) -> ()  [unwired: 9 in, 1 out]
  n161 = call <vilib>:"DestroyMessageQueue.vi"("error in (no error)"=w7, "Message Queue in"=w2) -> ()  [unwired: 9 in, 1 out]
